vi "Access Scope Example.vi"() -> ()   [LabVIEW 2020]
doc: "This example demonstrates public, private, and protected access scope for LabVIEW classes.\n\nRefer to the LabVIEW Help for more information about LabVIEW object-oriented programming."
uses:
  Widget Test Results/Widget Test Results.lvclass
  Test Results/Test Results Base Class.lvclass
panel:
  in  "widget identification":string="WTR 1"
  in  "time / date 1":timestamp=timestamp(3230370716.46 s since 1904-01-01)
  in  "result 1":bool
  in  "time / date 2":timestamp=timestamp(3230607139.8389997 s since 1904-01-01)
  in  "result 2":bool
  # "This example demonstrates public, private, and protected access scope for LabVIEW classes."
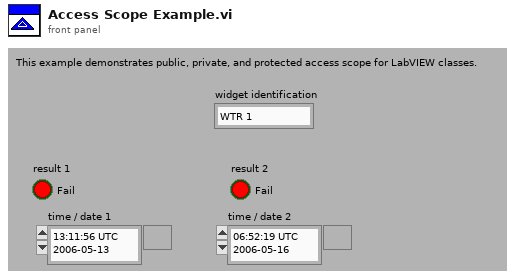
[diagram p1: front panel]
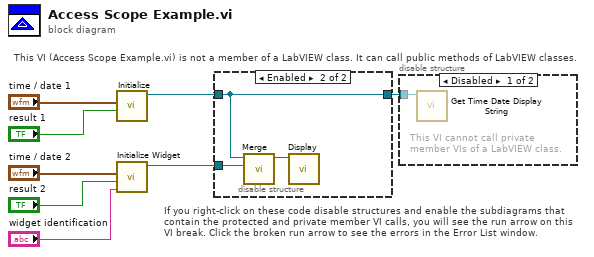
[diagram p0: block diagram]
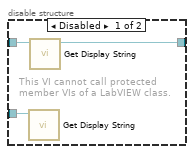
[diagram p3: hidden frame]
diagram:
  # "If you right-click on these code disable structures and enable the subdiagrams that contain the protected and private member VI calls, you will see the run arrow on this VI break. Click the broken run arrow to see the errors in the Error List window."
  # "This VI (Access Scope Example.vi) is not a member of a LabVIEW class. It can call public methods of LabVIEW classes."
  n1 = call "Initialize.vi"("result"="result 1", "time/date"="time / date 1") -> ("Test Results"=w3:refnum<class "Test Results Base Class.lvclass">)  [unwired: 9 in]
  n2 = call "Initialize Widget.vi"("widget identification"="widget identification", "result"="result 2", "time / date"="time / date 2") -> ("widget test results out"=w1:refnum<class "Widget Test Results.lvclass">)  [unwired: 8 in]
  n3 = disable-structure shown="Enabled" {
    disable-tunnel: w3 -> [w11 w14]
    disable-tunnel: [w10 w14] -> w2
    disable-tunnel: w1 -> [w9 w13]
    frame Disabled {
      # "This VI cannot call protected\nmember VIs of a LabVIEW class."
      n4 = call-dynamic "Get Display String.vi"("widget test\nresults in"=w9) -> ()  [unwired: 8 in, 3 out]
      n5 = call-dynamic "Get Display String.vi"("test\nresults in"=w11) -> ("test results out"=w10:refnum<class "Test Results Base Class.lvclass">)  [unwired: 8 in, 2 out]
    }
    frame Enabled {
      n6 = call "Merge.vi"("Test Results 2"=w13, "Test Results 1"=w14) -> ("Merged\nTest Results"=w12:refnum<class "Test Results Base Class.lvclass">)  [unwired: 8 in, 1 out]
      n7 = call "Display.vi"("Test Results"=w12) -> ()  [unwired: 10 in, 1 out]
    }
  }
  n8 = disable-structure shown="Disabled" {
    disable-tunnel: w2 -> [w15 _]
    frame Disabled {
      # "This VI cannot call private\nmember VIs of a LabVIEW class."
      n9 = call "Get Time Date Display String.vi"("test\n results in"=w15) -> ()  [unwired: 8 in, 3 out]
    }
    frame Enabled {
    }
  }
